vi "sub_status_transaction.vi"(8 "ERROR IN":errorcluster, 9 "RESULT":bool, 10 "MODE":u16(ring) items=["BEGIN", "RESULT"], 11 "TRANSACTION REF IN":refnum<vi>) -> (0 "ERROR OUT":errorcluster, 3 "TRANSACTION REF OUT":refnum<vi>)   [LabVIEW 2018]
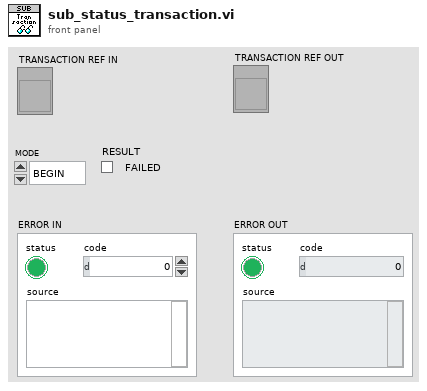
[diagram p1: front panel]
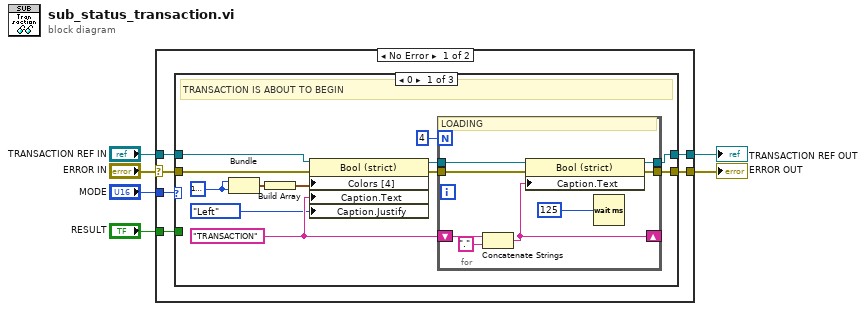
[diagram p0: block diagram]
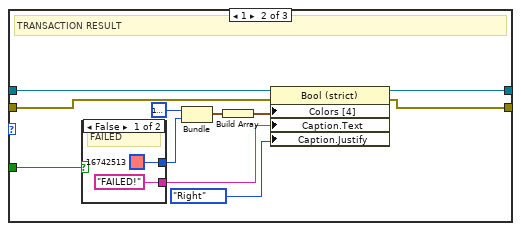
[diagram p2: hidden frame]
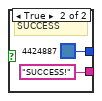
[diagram p3: hidden frame]
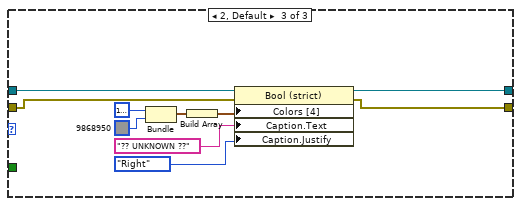
[diagram p4: hidden frame]
diagram:
  n1 = case shown="No Error" "ERROR IN" {
    selector: "ERROR IN" -> [w9 w58]
    tunnel: "TRANSACTION REF IN" -> [w12 w59]
    tunnel: [w11 w59] -> w5
    tunnel: [w10 w58] -> w4
    tunnel: "MODE" -> [w8 _]
    tunnel: "RESULT" -> [w7 _]
    frame No Error {
      n2 = case shown="0" w8 {
        tunnel: w12 -> [w17 w37 w54]
        tunnel: [w15 w34 w51] -> w10
        tunnel: [w14 w36 w52] -> w11
        tunnel: w9 -> [w13 w35 w53]
        tunnel: w7 -> [_ w33 _]
        frame 0 {
          w20 = "TRANSACTION"
          w19 = u32 16777226
          # "TRANSACTION IS ABOUT TO BEGIN"
          n3 = Bundle(w19, w19) -> (w24:cluster{u32, u32})  [unwired: 1 in]
          n4 = Build Array(w24) -> (w23:cluster{u32, u32}[])
          n5 = property on="Property Node" class="Bool (strict)"(reference=w17, error in=w13, "Colors [4]"=w23, "Caption.Text"=w20, "Caption.Justify"=enum16{"Left", "Center", "Right"}."Left" ("Caption.Justification")) -> (reference out=w16:refnum<vi>, error out=w21:errorcluster)
          n6 = for {
            N: 4 -> [_]
            tunnel: w21 -> [w30]
            shift-right: [w27] -> _
            shift-left: w20 -> [w32]
            tunnel: [w29] -> w15
            tunnel: w16 -> [w26]
            tunnel: [w25] -> w14
            # "LOADING"
            n7 = Concatenate Strings(w32, "." ("string")) -> (w27:string)
            n8 = property on="Property Node" class="Bool (strict)"(reference=w26, error in=w30, "Caption.Text"=w27) -> (reference out=w25:refnum<vi>, error out=w29:errorcluster)
            n9 = Wait (ms)(milliseconds to wait=u32 125) -> ()  [unwired: 1 out]
          }
        }
        frame 1 {
          # "TRANSACTION RESULT"
          n10 = case shown="False" w33 {
            tunnel: ["FAILED!" "SUCCESS!"] -> w40
            tunnel: [u32 16742513 u32 4424887] -> w41
            frame False {
              # "FAILED"
            }
            frame True {
              # "SUCCESS"
            }
          }
          n11 = Bundle(u32 16777226, w41) -> (w42:cluster{u32, u32})  [unwired: 1 in]
          n12 = Build Array(w42) -> (w43:cluster{u32, u32}[])
          n13 = property on="Property Node" class="Bool (strict)"(reference=w37, error in=w35, "Colors [4]"=w43, "Caption.Text"=w40, "Caption.Justify"=enum16{"Left", "Center", "Right"}."Right" ("Caption.Justification")) -> (reference out=w36:refnum<vi>, error out=w34:errorcluster)
        }
        frame 2, Default {
          n14 = Bundle(u32 16777226, u32 9868950) -> (w56:cluster{u32, u32})  [unwired: 1 in]
          n15 = Build Array(w56) -> (w57:cluster{u32, u32}[])
          n16 = property on="Property Node" class="Bool (strict)"(reference=w54, error in=w53, "Colors [4]"=w57, "Caption.Text"="?? UNKNOWN ??", "Caption.Justify"=enum16{"Left", "Center", "Right"}."Right" ("Caption.Justification")) -> (reference out=w52:refnum<vi>, error out=w51:errorcluster)
        }
      }
    }
    frame Error {
    }
  }
  "TRANSACTION REF OUT" <- w5
  "ERROR OUT" <- w4
